vi "Read Waveform Data.vi"(8 "error in (no error)":errorcluster, 10 "acq duration (s)":dbl, 11 "task":T1) -> (0 "error out":errorcluster, 2 "waveforms":waveform(dbl)[](array[waveform]), 3 "task":T1)   [LabVIEW 2022 SP3, in "Combo Digital Audio API.lvlib"]
uses:
  Combo Digital Audio API.lvlib
  task.ctl
  controls/input type.ctl
  task conversion/From PDM task.vi
  <vilib>/PDM Acquisition Toolkit/host/API/Public/Read/Read PCM Input Waveform.vi
  task conversion/From PCM task.vi
  task conversion/To PCM task.vi
  task conversion/To PDM task.vi
  <vilib>/PDM Acquisition Toolkit/host/API/Public/Read/Read PCM Waveform.vi
  <vilib>/PDM Acquisition Toolkit/host/API/PDM Acquisition Toolkit.lvlib
  task conversion/DAAG task conversion.lvlib
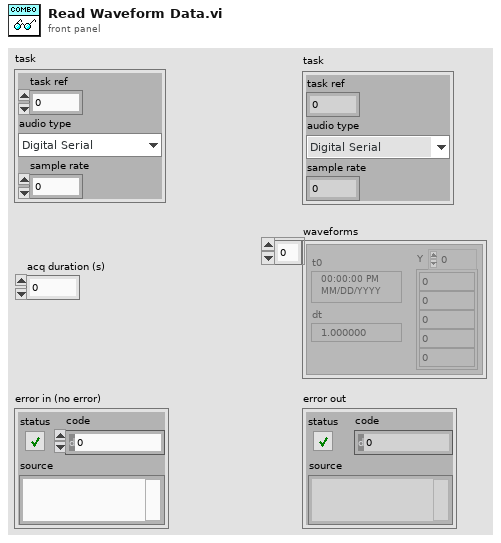
[diagram p1: front panel]
types:
  T1 = typedef "Combo Digital Audio API.lvlib/task.ctl" = cluster{"task ref":u64, "audio type":T2, "sample rate":dbl}
  T2 = typedef "input type.ctl" = enum32{"Digital Serial", "PDM"}
  T3 = typedef "PDM Acquisition Class Library.lvlib/PCM Input Task.lvclass/DVR PCM Input Task.ctl" = refnum<data-value>
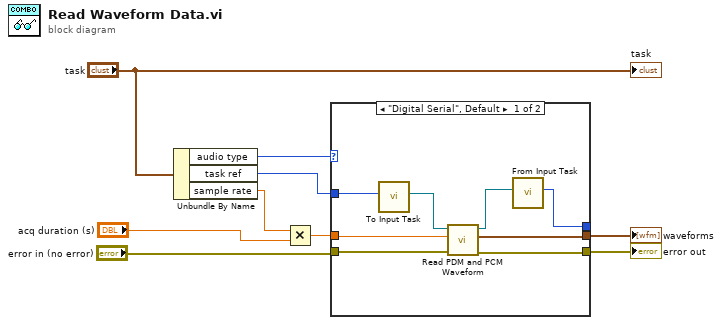
[diagram p0: block diagram]
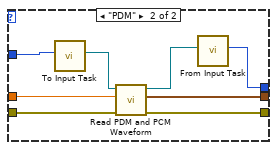
[diagram p2: hidden frame]
diagram:
  n1 = Unbundle By Name("task") -> ("audio type"=w6:T2, "task ref"=w5:u64, "sample rate"=w2:dbl)
  n2 = Multiply(x=w2, y="acq duration (s)") -> (x*y=w3:dbl)
  n3 = case shown="\"Digital Serial\", Default" w6 {
    tunnel: "error in (no error)" -> [w17 w25]
    tunnel: w3 -> [w16 w24]
    tunnel: [w14 w23] -> w8
    tunnel: [w15 w22] -> w7
    tunnel: w5 -> [w13 w21]
    tunnel: [w10 w18] -> _
    frame "Digital Serial", Default {
      n4 = call-poly "To Input Task.vi"("task"=w13) -> ("PCM task"=w12:T3)  [unwired: 10 in]
      n5 = call-poly <vilib>:"Read PDM and PCM Waveform.vi"("error in"=w17, "words per channel"=w16, "PCM input task In"=w12) -> ("error out"=w14:errorcluster, "PCM waveforms"=w15:waveform(dbl)[], "PCM input task out"=w11:T3)  [unwired: 3 in, 3 out]
      n6 = call-poly "From Input Task.vi"("PCM input task"=w11) -> ("task"=w10:u64)  [unwired: 10 in]
    }
    frame "PDM" {
      n7 = call-poly "To Input Task.vi"("task"=w21) -> ("PDM task"=w20:refnum<data-value>)  [unwired: 10 in]
      n8 = call-poly <vilib>:"Read PDM and PCM Waveform.vi"("error in"=w25, "samples per channel"=w24, "PDM input task in"=w20) -> ("error out"=w23:errorcluster, "PCM waveforms"=w22:waveform(dbl)[], "PDM input task out"=w19:refnum<data-value>)  [unwired: 5 in, 1 out]
      n9 = call-poly "From Input Task.vi"("PDM input task"=w19) -> ("task"=w18:u64)  [unwired: 10 in]
    }
  }
  "error out" <- w8
  "waveforms" <- w7
  "task" <- "task"
